vi "SpreadsheetFGV2_Improvements.vi"(0 "Student ID":i32, 1 "FGV Control":T3=enum."Init", 2 "Camera Name":refnum<k21> caption="IMAQdx Session", 11 "Error In":errorcluster) -> (3 "Time Stamp Out":timestamp, 4 "Message":string, 6 "Names":string[](array[string]), 8 "Output 2D Data":string[][](array[string]), 10 "Checked In?":bool, 12 "Cat Points":i32, 13 "Image Out":T1(plugin-control), 14 "Elapsed Time":dbl, 15 "Error Out":errorcluster)   [LabVIEW 2013]
uses:
  Controls/CSVFGVStates.ctl
  <vilib>/userdefined/High Color/IMAQdx.ctl
  Controls/SpreadsheetColumns.ctl
  <vilib>/Utility/file.llb/Write To Spreadsheet File (string).vi
  <vilib>/Utility/file.llb/Read From Spreadsheet File (string).vi
  <vilib>/vision/driver/NI_Vision_Acquisition_Software.lvlib
panel:
  out "Session Out":T2
  out "Checked In":string
  out "all rows":string[][](array[string])
  in  "Replacement":string
  in  "Student Names":i32(listbox)
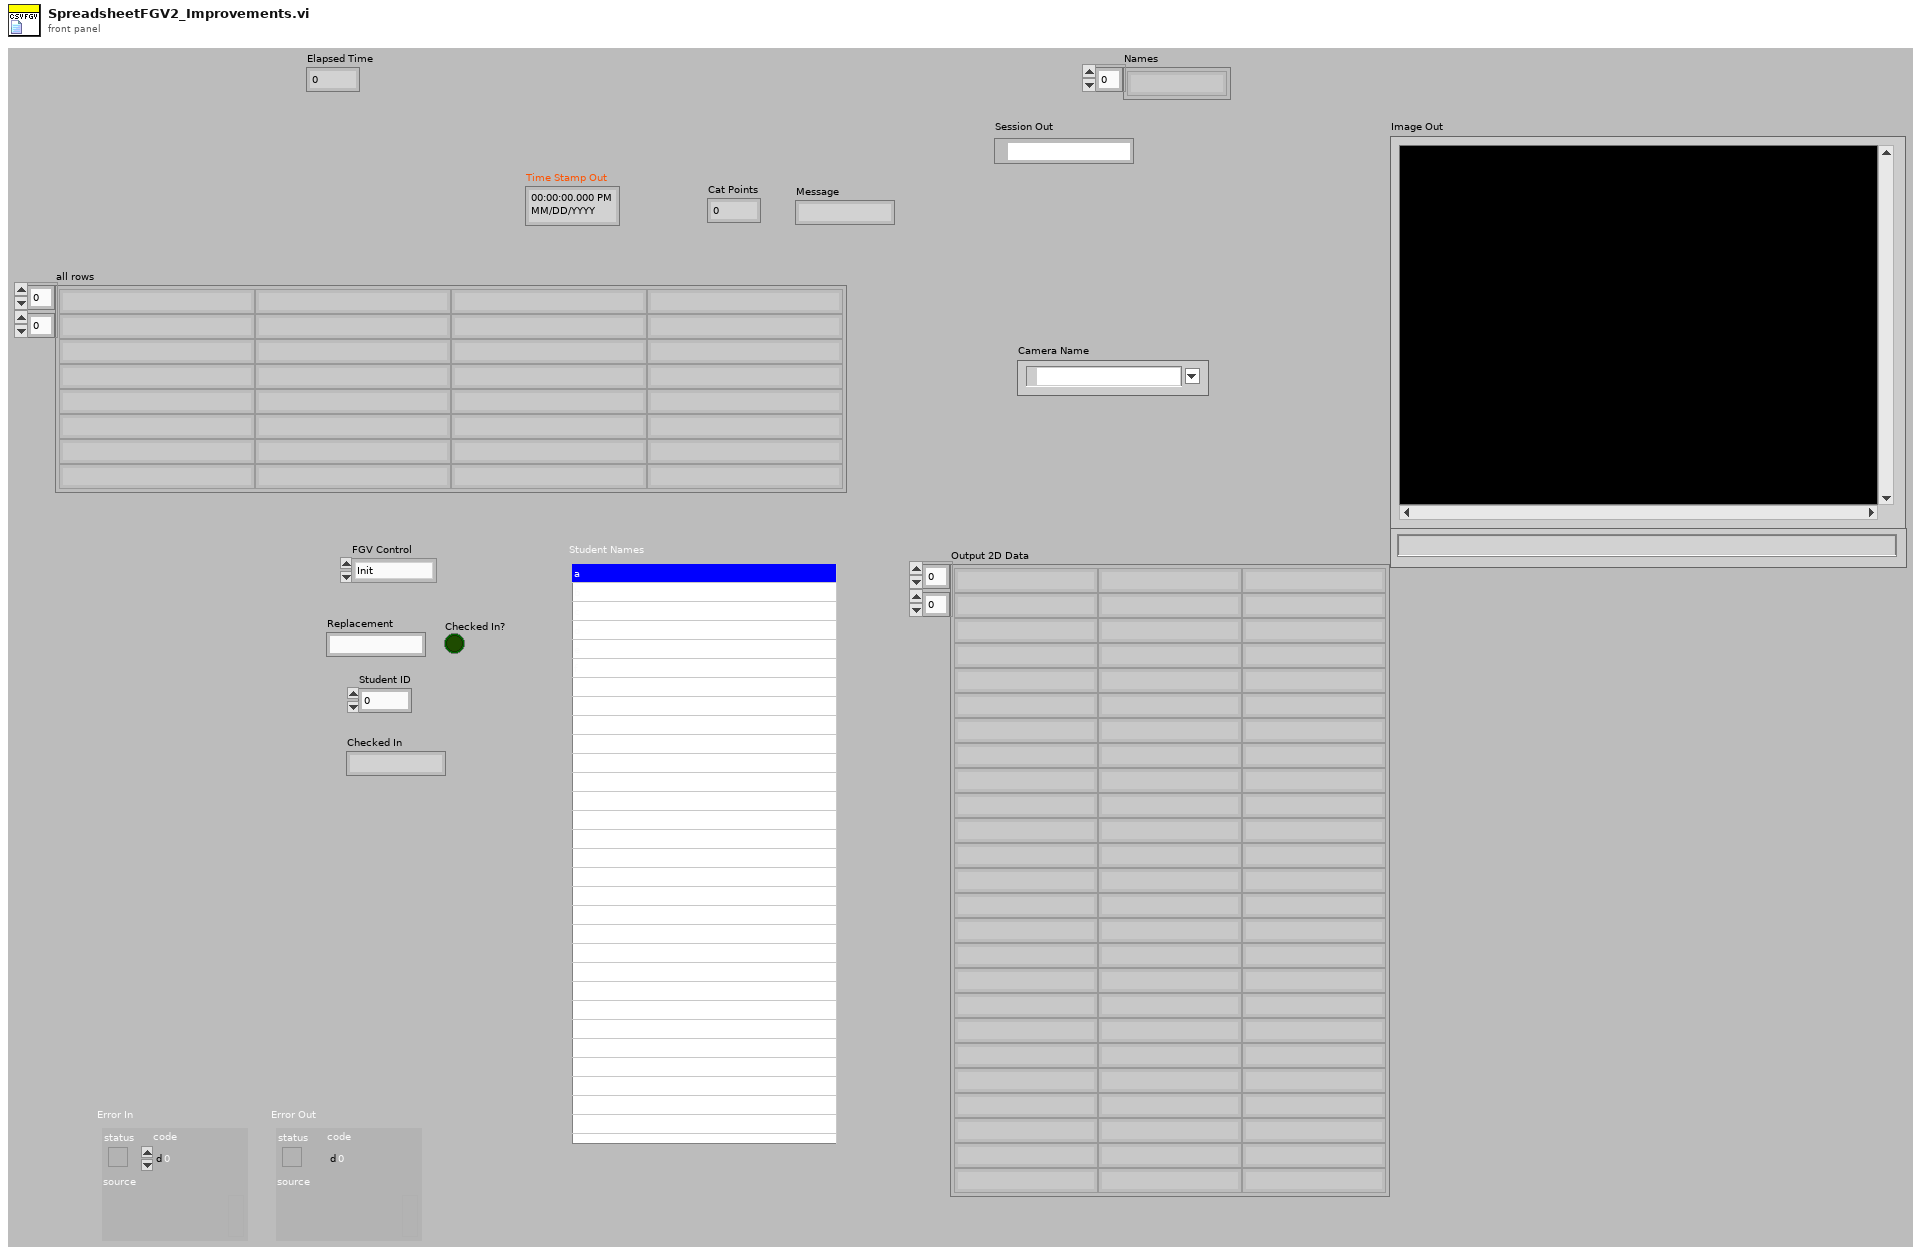
[diagram p1: front panel]
types:
  T1 = typedef "IMAQ Image.ctl" = refnum<image>
  T2 = typedef "IMAQdx.ctl" = refnum<k21>
  T3 = typedef "CSVFGVStates.ctl" = enum16{"Quit", "Init", "Sort", "Check In", "Check Out", "Check Status", "Read CSV", "Close Out"}
  T4 = typedef "SpreadsheetColumns.ctl" = enum16{"Email", "CheckIn", "CheckOut", "Checkin Flag", "Hours", "Minutes", "Seconds", "Total Seconds", "Cat Points"}
  T5 = cluster{"Checkin Flag":T4, "Check In":T4, "Hours":T4, "Minutes":T4, "Seconds":T4, "Check Out":T4, "Email":T4, "Total Seconds":T4}
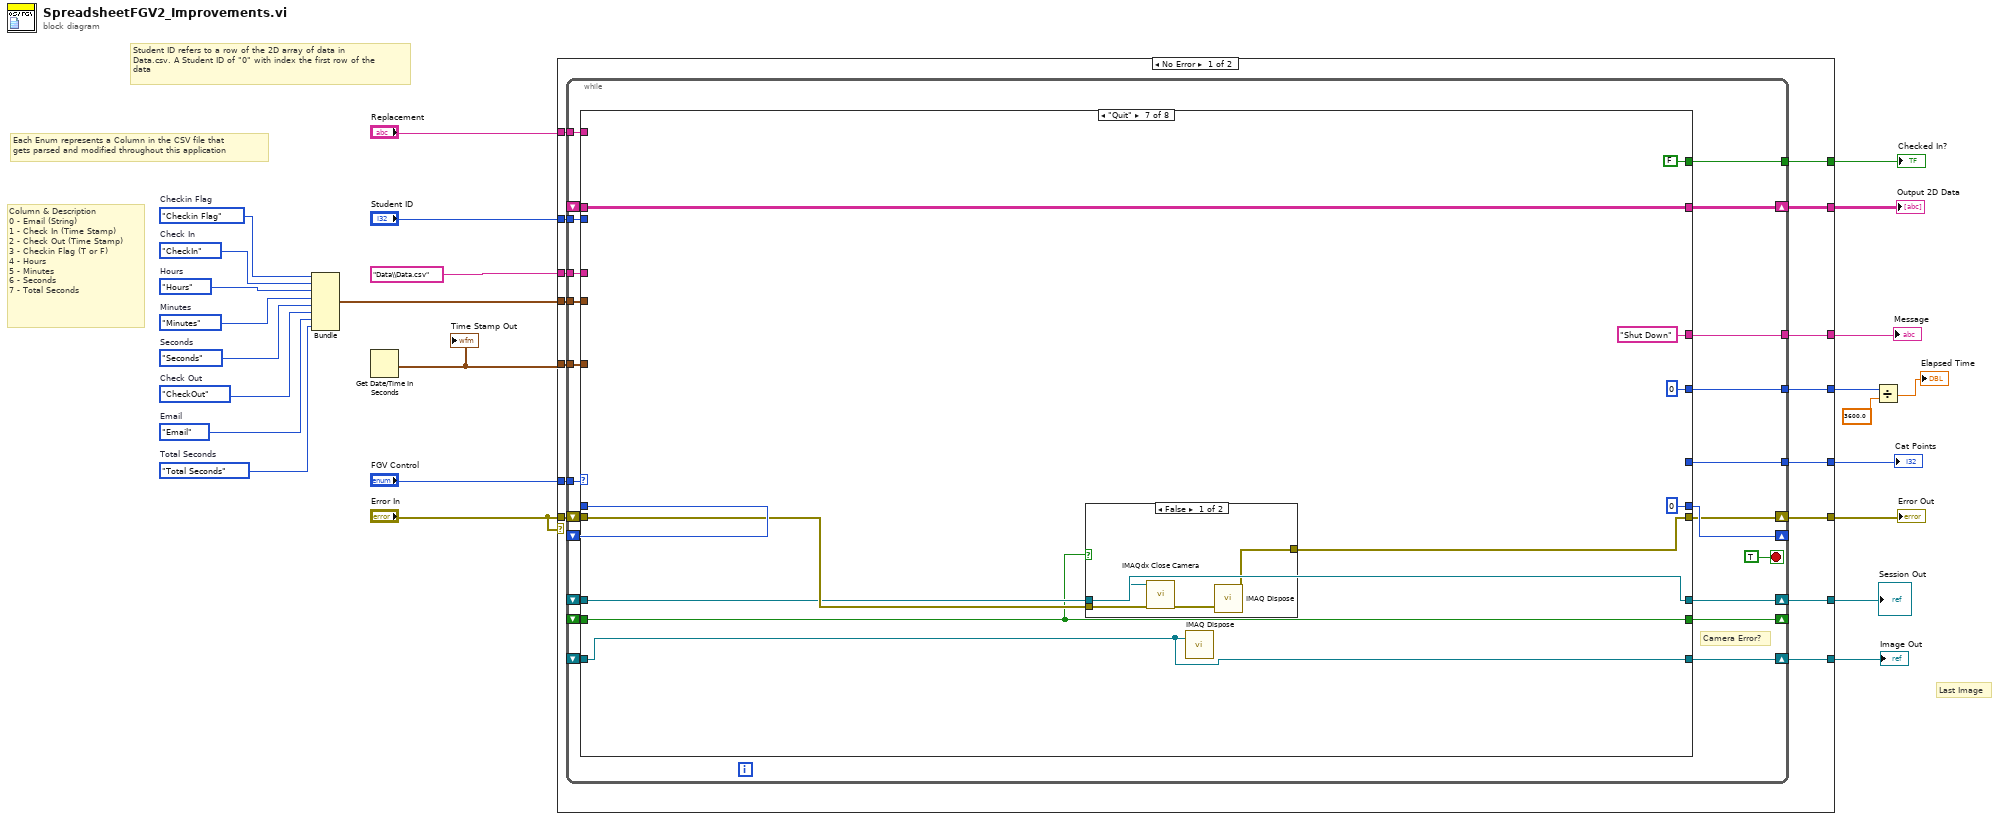
[diagram p0: block diagram]
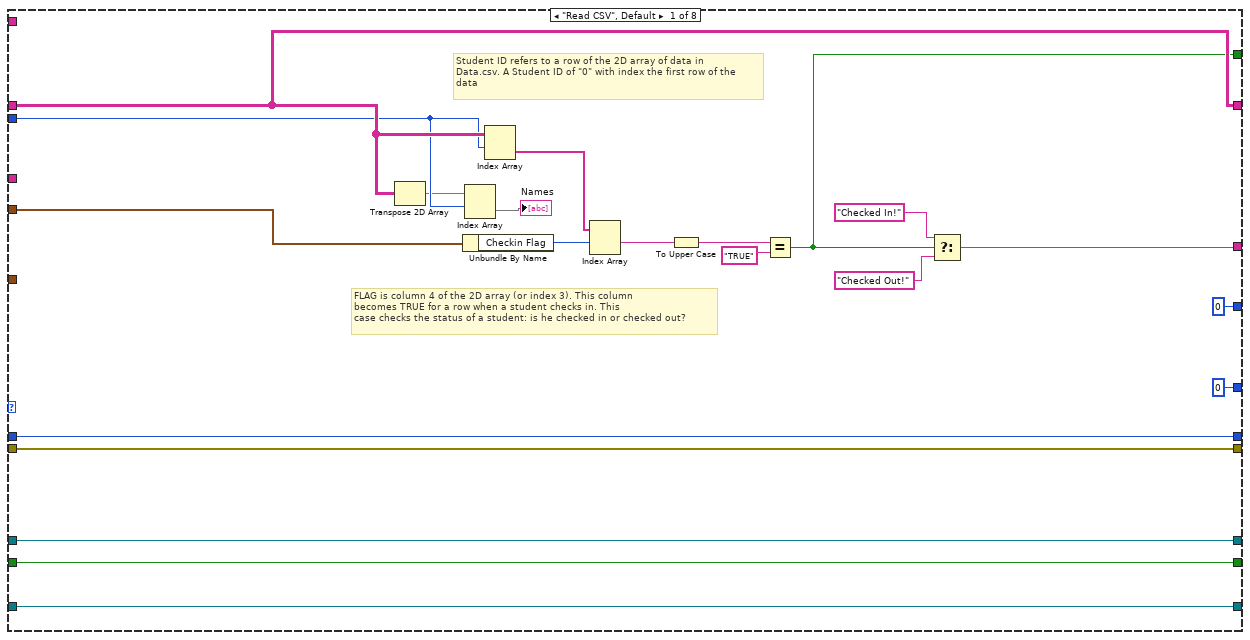
[diagram p2: hidden frame]
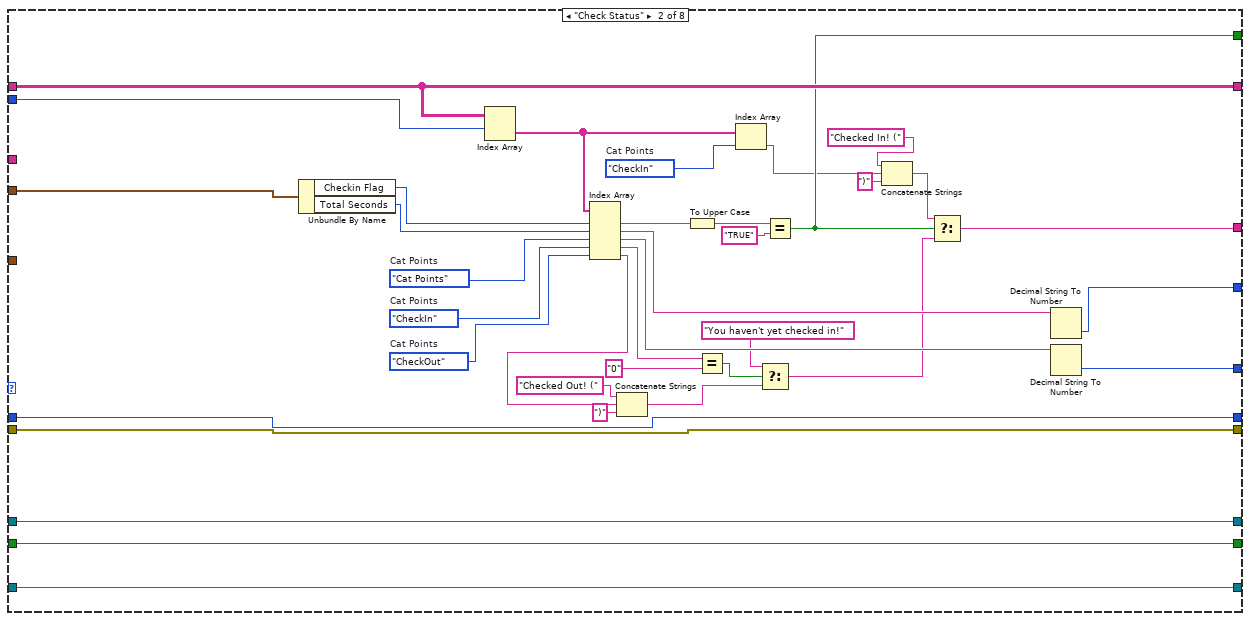
[diagram p3: hidden frame]
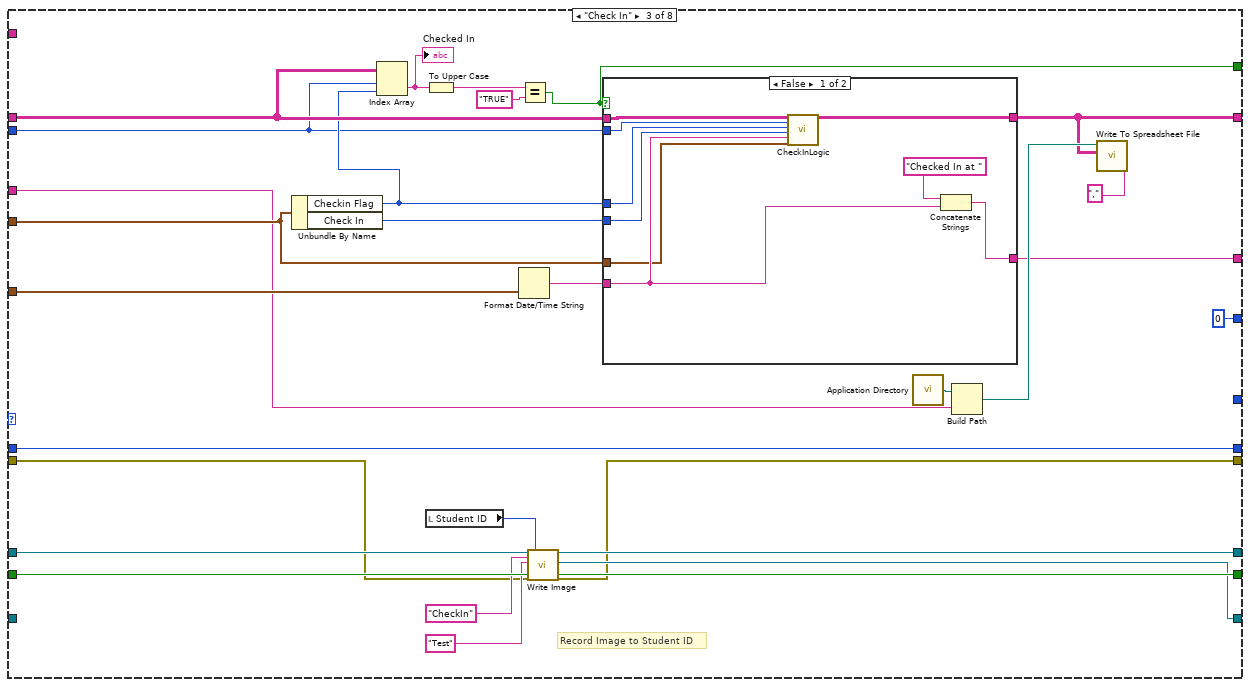
[diagram p4: hidden frame]
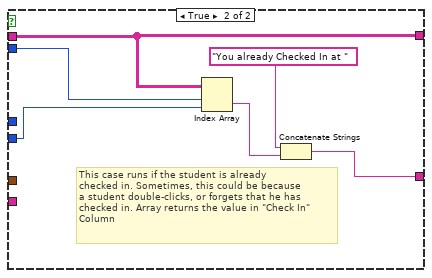
[diagram p5: hidden frame]
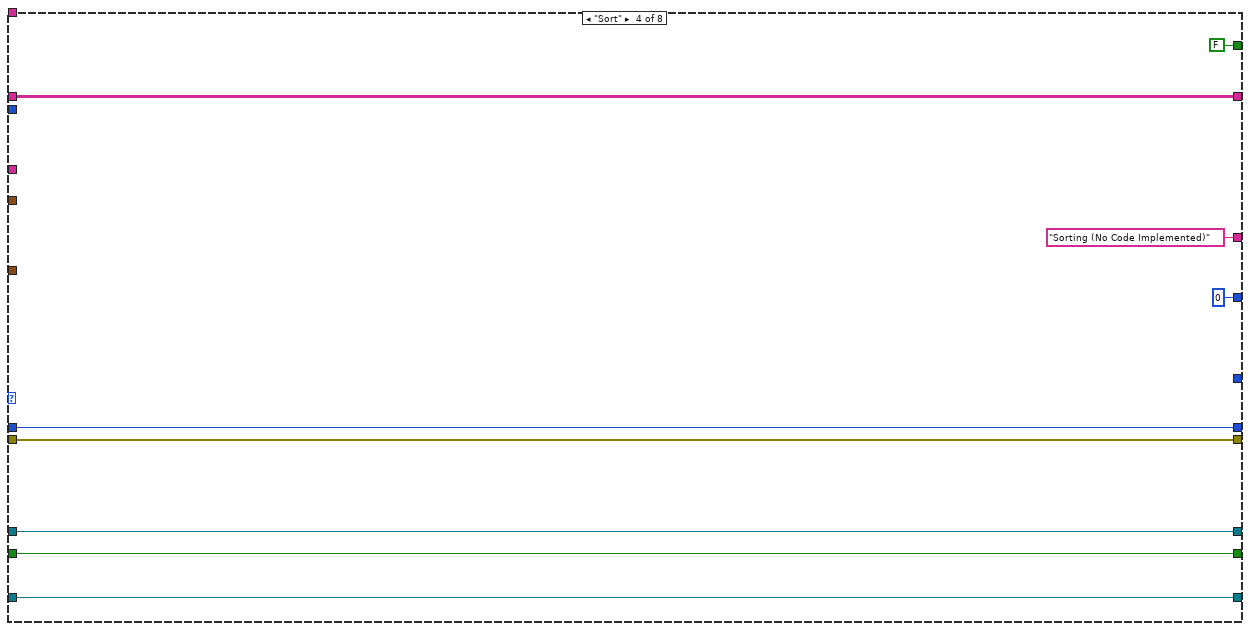
[diagram p6: hidden frame]
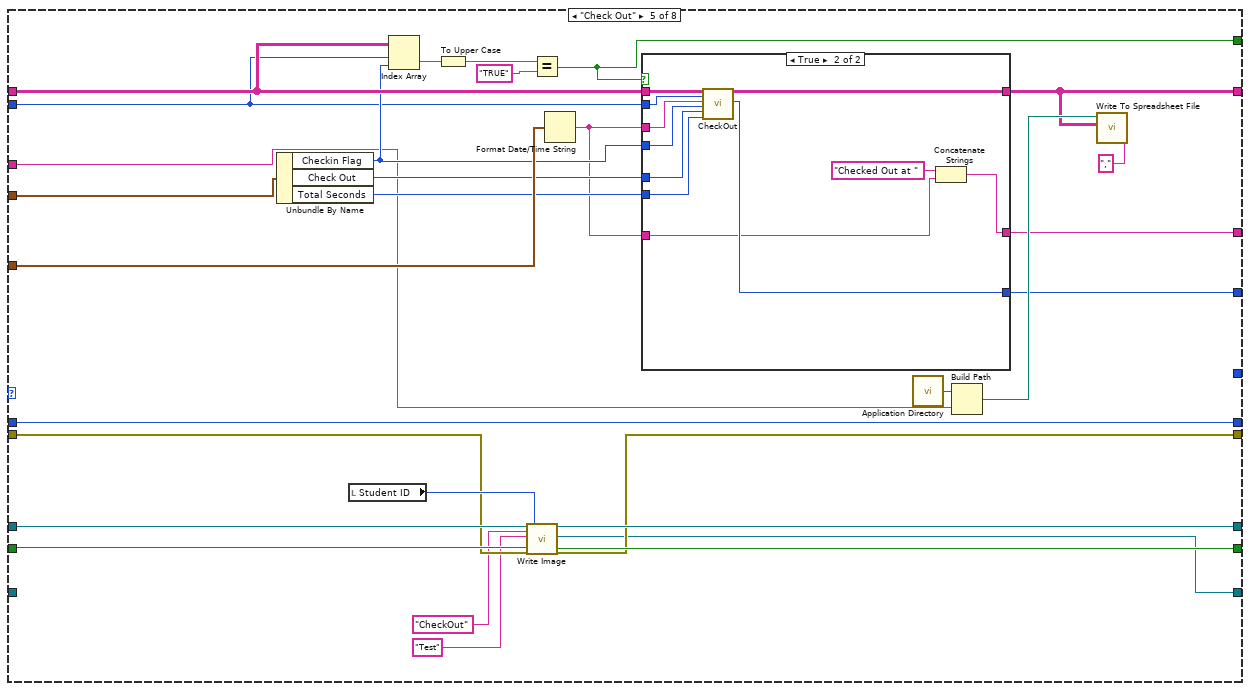
[diagram p7: hidden frame]
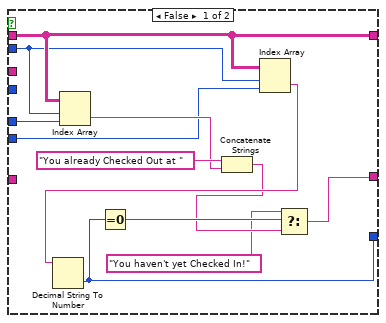
[diagram p8: hidden frame]
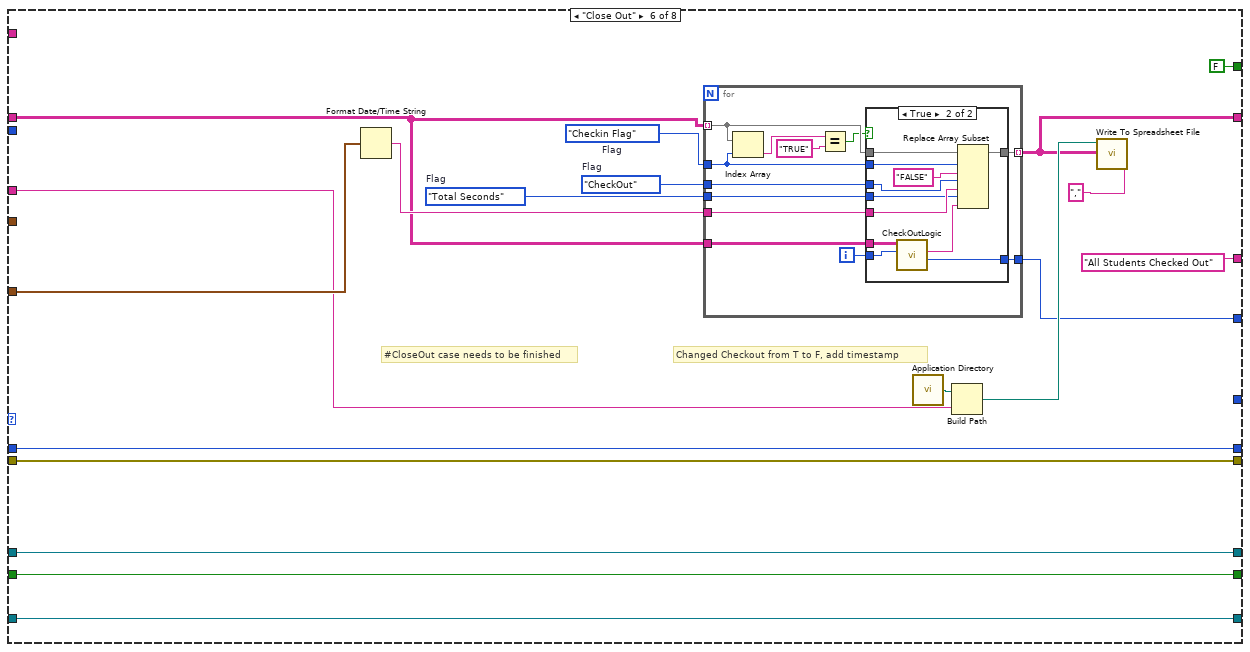
[diagram p9: hidden frame]
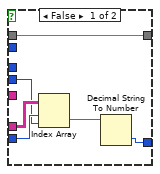
[diagram p10: hidden frame]
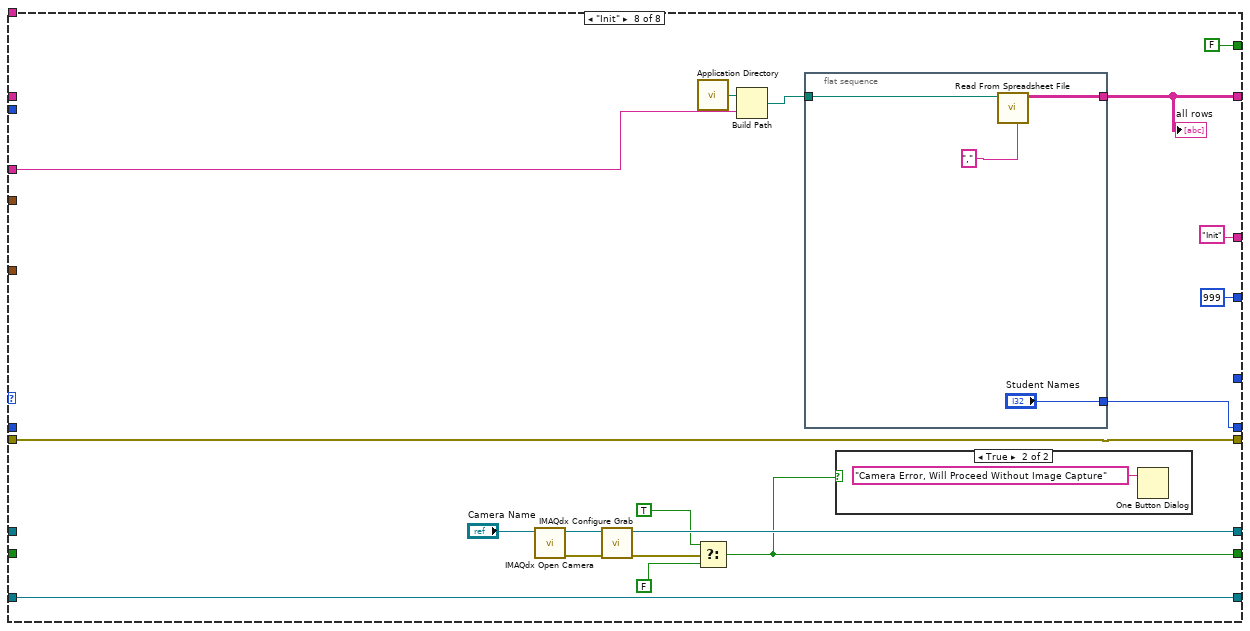
[diagram p12: hidden frame]
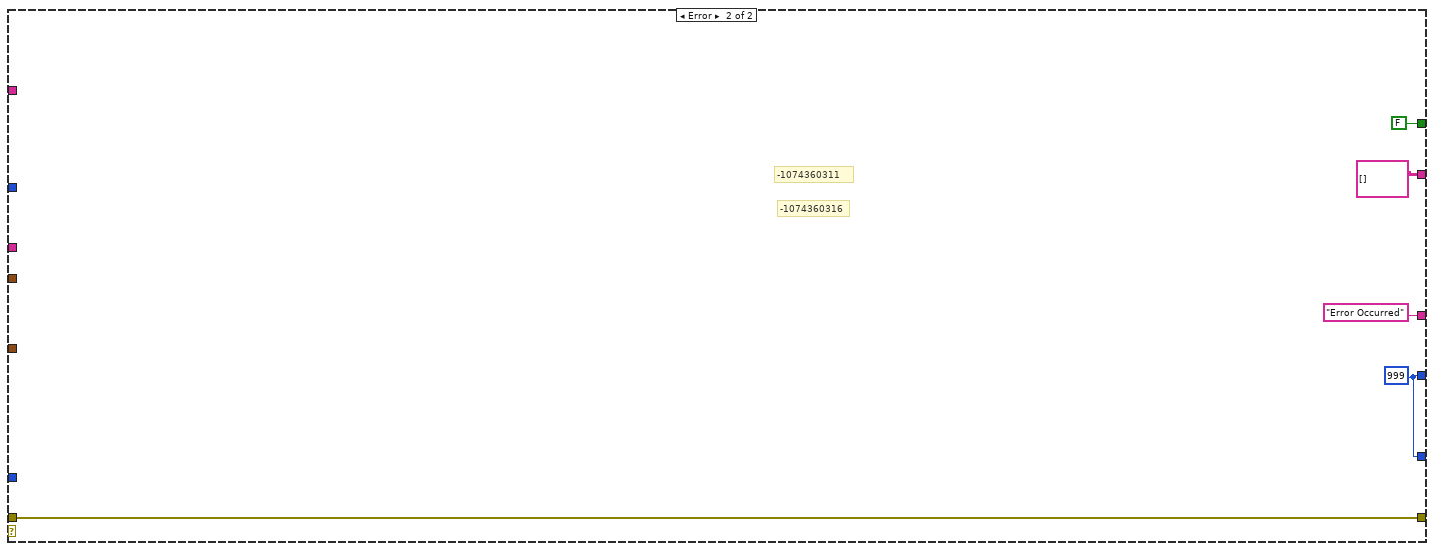
[diagram p14: hidden frame]
diagram:
  w10 = SpreadsheetColumns."Total Seconds"  # Total Seconds
  w11 = SpreadsheetColumns."Email"  # Email
  w12 = SpreadsheetColumns."CheckOut"  # Check Out
  w14 = SpreadsheetColumns."Seconds"  # Seconds
  w15 = SpreadsheetColumns."Minutes"  # Minutes
  w16 = SpreadsheetColumns."Hours"  # Hours
  w18 = SpreadsheetColumns."Checkin Flag"  # Checkin Flag
  w17 = SpreadsheetColumns."CheckIn"  # Check In
  # "Student ID refers to a row of the 2D array of data in \nData.csv. A Student ID of \"0\" with index the first row of the\ndata"
  # "Each Enum represents a Column in the CSV file that\ngets parsed and modified throughout this application"
  # "Last Image"
  # "Column & Description\n0 - Email (String)\n1 - Check In (Time Stamp)\n2 - Check Out (Time Stamp)\n3 - Checkin Flag (T or F)\n4 - Hours\n5 - Minutes\n6 - Seconds\n7 - Total Seconds"
  n1 = Bundle("Checkin Flag"=w18, "Check In"=w17, "Hours"=w16, "Minutes"=w15, "Seconds"=w14, "Check Out"=w12, "Email"=w11, "Total Seconds"=w10) -> (w13:T5)  [unwired: 1 in]
  n2 = Get Date/Time In Seconds() -> (seconds since 1Jan1904=w7:timestamp)
  "Time Stamp Out" <- w7
  n3 = case shown="No Error" "Error In" {
    tunnel: "FGV Control" -> [w40 _]
    tunnel: "Error In" -> [w38 w312]
    tunnel: [w39 w312] -> w23
    tunnel: "Student ID" -> [w37 _]
    tunnel: w7 -> [w36 _]
    tunnel: "Replacement" -> [w35 _]
    tunnel: [w34 FALSE] -> w9
    tunnel: [w33 string[][] [] ("all rows")] -> w20
    tunnel: [w32 "Error Occurred" ("date/time string")] -> w19
    tunnel: [w31 w313] -> w4
    tunnel: w13 -> [w30 _]
    tunnel: "Data\\Data.csv" ("name or relative path") -> [w29 _]
    tunnel: [w28 w313] -> w6
    tunnel: [w27 _] -> w2
    tunnel: [w26 _] -> w1
    frame No Error {
      n4 = while {
        shift-right: [w54] -> w33
        shift-left: _ -> [w49]
        tunnel: w40 -> [w62]
        shift-right: [w61] -> _
        shift-left: _ -> [w60]
        shift-right: [w59] -> w39
        shift-left: w38 -> [w58]
        tunnel: w37 -> [w57]
        tunnel: w36 -> [w56]
        tunnel: w35 -> [w55]
        tunnel: [w53] -> w34
        tunnel: [w52] -> w32
        tunnel: [w51] -> w31
        tunnel: w30 -> [w50]
        tunnel: w29 -> [w48]
        tunnel: [w47] -> w28
        shift-right: [w46] -> w27
        shift-left: _ -> [w45]
        shift-right: [w44] -> w26
        shift-left: _ -> [w43]
        shift-right: [w42] -> _
        shift-left: _ -> [w41]
        stop <- TRUE stop-if-true
        # "Camera Error?"
        n5 = case shown="\"Quit\"" w62 {
          tunnel: w49 -> [w74 w115 w138 w168 w193 w230 w283 _]
          tunnel: [w83 w120 w147 w172 w200 w241 0 ("Student Names") w305] -> w61
          tunnel: w60 -> [w83 w120 w147 w172 w200 w241 _ _]
          tunnel: [w84 w121 w122 w173 w177 w243 w278 w293] -> w59
          tunnel: w58 -> [w84 w121 w123 w173 w178 w243 w277 w293]
          tunnel: w57 -> [w73 w111 w131 _ w183 _ _ _]
          tunnel: w56 -> [_ _ w140 _ w198 w239 _ _]
          tunnel: w55 -> [_ _ _ _ _ _ _ _]
          tunnel: [w74 w115 w133 w168 w197 w238 w283 w299] -> w54
          tunnel: [w70 w112 w137 FALSE w187 FALSE FALSE FALSE] -> w53
          tunnel: [w75 w116 w141 "Sorting (No Code Implemented)" ("date/time string") w192 "All Students Checked Out" ("date/time string") "Shut Down" ("date/time string") "Init" ("date/time string")] -> w52
          tunnel: [0 ("Elapsed Seconds") w108 0 ("Elapsed Seconds") 0 ("Elapsed Seconds") w191 w229 0 ("Elapsed Seconds") 999 ("Elapsed Seconds")] -> w51
          tunnel: w50 -> [w69 w114 w136 _ w190 _ _ _]
          tunnel: w48 -> [_ _ w135 _ w185 w234 _ w300]
          tunnel: [0 w105 _ _ _ _ _ _] -> w47
          tunnel: [w66 w87 w125 w167 w180 w228 w276 w295] -> w46
          tunnel: w45 -> [w66 w87 w130 w167 w181 w228 w276 _]
          tunnel: [w65 w86 w124 w166 w176 w227 w274 w294] -> w44
          tunnel: w43 -> [w65 w86 _ w166 _ w227 w274 w294]
          tunnel: [w64 w85 w129 w165 w179 w226 w275 w289] -> w42
          tunnel: w41 -> [w64 w85 w129 w165 w179 w226 w275 _]
          frame "Read CSV", Default {
            # "FLAG is column 4 of the 2D array (or index 3). This column\nbecomes TRUE for a row when a student checks in. This\ncase checks the status of a student: is he checked in or checked out?"
            # "Student ID refers to a row of the 2D array of data in \nData.csv. A Student ID of \"0\" with index the first row of the\ndata"
            n6 = Transpose 2D Array(2D array=w74) -> (transposed array=w72:string[][])
            n7 = Unbundle By Name(w69) -> ("Checkin Flag"=w68:T4)
            n8 = Index Array(array=w72, index (row)=w73) -> (element=→"Names":string[])  [unwired: 1 in]
            n9 = Index Array(array=w74, index (row)=w73) -> (element=w78:string[])  [unwired: 1 in]
            n10 = Index Array(array=w78, index #1=w68) -> (element #1=w81:string)  [unwired: 1 in, 1 out]
            n11 = To Upper Case(1:w81) -> (0:w80:string)
            n12 = Equal?(x=w80, y="TRUE") -> (x = y?=w70:bool)
            n13 = Select(t="Checked In!" ("y"), s=w70, f="Checked Out!" ("y")) -> (s? t:f=w75:string)
          }
          frame "Check Status" {
            w93 = SpreadsheetColumns."CheckIn"  # Cat Points
            w92 = SpreadsheetColumns."CheckOut"  # Cat Points
            w104 = SpreadsheetColumns."CheckIn"  # Cat Points
            w107 = SpreadsheetColumns."Cat Points"  # Cat Points
            n14 = Unbundle By Name(w114) -> ("Checkin Flag"=w113:T4, "Total Seconds"=w110:T4)
            n15 = Index Array(array=w115, index (row)=w111) -> (element=w94:string[])  [unwired: 1 in]
            n16 = Index Array(array=w94, index #1=w113, index #2=w110, index #3=w107, index #4=w104, index #5=w92) -> (element #1=w119:string, element #2=w109:string, element #3=w106:string, element #4=w103:string, element #5=w96:string)
            n17 = Concatenate Strings("Checked Out! (" ("y"), w96, ")" ("string")) -> (w97:string)
            n18 = To Upper Case(1:w119) -> (0:w118:string)
            n19 = Equal?(x=w103, y="0") -> (x = y?=w101:bool)
            n20 = Index Array(array=w94, index=w93) -> (element=w90:string)
            n21 = Select(t="You haven't yet checked in!", s=w101, f=w97) -> (s? t:f=w100:string)
            n22 = Equal?(x=w118, y="TRUE") -> (x = y?=w112:bool)
            n23 = Concatenate Strings("Checked In! (" ("y"), w90, ")" ("string")) -> (w88:string)
            n24 = Select(t=w88, s=w112, f=w100) -> (s? t:f=w116:string)
            n25 = Decimal String To Number(string=w109) -> (number=w108:i32)  [unwired: 2 in, 1 out]
            n26 = Decimal String To Number(string=w106) -> (number=w105:i32)  [unwired: 2 in, 1 out]
          }
          frame "Check In" {
            # "Record Image to Student ID"
            n27 = Unbundle By Name(w136) -> ("Checkin Flag"=w134:T4, "Check In"=w139:T4)
            n28 = Index Array(array=w138, index (row)=w131, index (col)=w134) -> (element=w144:string)
            "Checked In" <- w144
            n29 = To Upper Case(1:w144) -> (0:w143:string)
            n30 = local read "Student ID"() -> (w128:i32)
            n31 = Format Date/Time String(seconds (now)=w140) -> (date/time string=w145:string)  [unwired: 2 in]
            n32 = Equal?(x=w143, y="TRUE") -> (x = y?=w137:bool)
            n33 = call "Write Image.vi"("Session In"=w130, "Folder"="CheckIn", "Temp Image Name"="Test" ("Image Name"), "Camera Missing?"=w129, "Error In"=w123, "Student ID"=w128) -> ("Session Out"=w125:T2, "Image Out"=w124:T1, "Error Out"=w122:errorcluster)  [unwired: 11 in]
            n34 = case shown="False" w137 {
              tunnel: w145 -> [w151 _]
              tunnel: [w155 w164] -> w133
              tunnel: w131 -> [w154 w163]
              tunnel: w138 -> [w156 w164]
              tunnel: [w157 w160] -> w141
              tunnel: w134 -> [w153 _]
              tunnel: w139 -> [w152 w159]
              tunnel: w136 -> [w150 _]
              frame False {
                n35 = call "CheckInLogic.vi"("all rows in"=w156, "Student ID"=w154, "Checkin Flag"=w153, "Check In"=w152, "date/time string"=w151, "Time Cluster"=w150) -> ("all rows out"=w155:string[][])  [unwired: 13 in]
                n36 = Concatenate Strings("Checked In at " ("String"), w151) -> (w157:string)
              }
              frame True {
                # "This case runs if the student is already \nchecked in. Sometimes, this could be because\na student double-clicks, or forgets that he has \nchecked in. Array returns the value in \"Check In\" \nColumn"
                n37 = Index Array(array=w164, index (row)=w163, index (col)=w159) -> (element=w161:string)
                n38 = Concatenate Strings("You already Checked In at " ("delimiter (\\t)"), w161) -> (w160:string)
              }
            }
            n39 = call <vilib>:"Application Directory.vi"() -> ("Application Directory"=w149:path)
            n40 = Build Path(base path=w149, name or relative path=w135) -> (appended path=w148:path)
            n41 = call-poly <vilib>:"Write To Spreadsheet File.vi"("delimiter (\\t)"="," ("delimiter (\\t)"), "2D data"=w133, "file path (dialog if empty)"=w148) -> ()  [unwired: 5 in, 1 out]
          }
          frame "Sort" {
          }
          frame "Check Out" {
            n42 = Unbundle By Name(w190) -> ("Checkin Flag"=w186:T4, "Check Out"=w188:T4, "Total Seconds"=w189:T4)
            n43 = local read "Student ID"() -> (w182:i32)
            n44 = Index Array(array=w193, index (row)=w183, index (col)=w186) -> (element=w196:string)
            n45 = To Upper Case(1:w196) -> (0:w195:string)
            n46 = call "Write Image.vi"("Session In"=w181, "Folder"="CheckOut", "Temp Image Name"="Test" ("Image Name"), "Camera Missing?"=w179, "Error In"=w178, "Student ID"=w182) -> ("Session Out"=w180:T2, "Image Out"=w176:T1, "Error Out"=w177:errorcluster)  [unwired: 11 in]
            n47 = Equal?(x=w195, y="TRUE") -> (x = y?=w187:bool)
            n48 = Format Date/Time String(seconds (now)=w198) -> (date/time string=w184:string)  [unwired: 2 in]
            n49 = case shown="True" w187 {
              tunnel: [w211 w222] -> w197
              tunnel: w183 -> [w210 w221]
              tunnel: w193 -> [w211 w223]
              tunnel: [w204 w225] -> w192
              tunnel: [w207 w216] -> w191
              tunnel: w189 -> [w209 w219]
              tunnel: w188 -> [w212 w220]
              tunnel: w186 -> [_ w218]
              tunnel: w184 -> [_ w217]
              tunnel: w184 -> [_ w215]
              frame False {
                n50 = Index Array(array=w211, index (row)=w210, index (col)=w212) -> (element=w213:string)
                n51 = Concatenate Strings("You already Checked Out at " ("string"), w213) -> (w205:string)
                n52 = Index Array(array=w211, index (row)=w210, index (col)=w209) -> (element=w208:string)
                n53 = Decimal String To Number(string=w208) -> (number=w207:i32)  [unwired: 2 in, 1 out]
                n54 = Equal To 0?(x=w207) -> (x = 0?=w206:bool)
                n55 = Select(t="You haven't yet Checked In!", s=w206, f=w205) -> (s? t:f=w204:string)
              }
              frame True {
                n56 = call "CheckOut.vi"("Student List In"=w223, "Student ID"=w221, "date/time string"=w217, "Checkin Flag"=w218, "Check Out"=w220, "Total Seconds"=w219) -> ("Student List Out"=w222:string[][], "Total Elapsed Time"=w216:i32)  [unwired: 12 in]
                n57 = Concatenate Strings("Checked Out at " ("string"), w215) -> (w225:string)
              }
            }
            n58 = call <vilib>:"Application Directory.vi"() -> ("Application Directory"=w202:path)
            n59 = Build Path(base path=w202, name or relative path=w185) -> (appended path=w201:path)
            n60 = call-poly <vilib>:"Write To Spreadsheet File.vi"("delimiter (\\t)"="," ("delimiter (\\t)"), "2D data"=w197, "file path (dialog if empty)"=w201) -> ()  [unwired: 5 in, 1 out]
          }
          frame "Close Out" {
            w231 = SpreadsheetColumns."Total Seconds"  # Flag
            w232 = SpreadsheetColumns."CheckOut"  # Flag
            w233 = SpreadsheetColumns."Checkin Flag"  # Flag
            # "#CloseOut case needs to be finished"
            # "Changed Checkout from T to F, add timestamp"
            n61 = Format Date/Time String(seconds (now)=w239) -> (date/time string=w236:string)  [unwired: 2 in]
            n62 = for {
              tunnel: [w256] -> w238 mode=indexing
              tunnel: w230 -> [w249] mode=indexing
              tunnel: w236 -> [w255]
              tunnel: w233 -> [w248]
              tunnel: w232 -> [w254]
              tunnel: w231 -> [w252]
              tunnel: w230 -> [w251]
              tunnel: [w250] -> w229
              i -> [w253]
              n63 = Index Array(array=w249, index=w248) -> (element=w247:string)
              n64 = Equal?(x=w247, y="TRUE") -> (x = y?=w245:bool)
              n65 = case shown="True" w245 {
                tunnel: [w262 w273] -> w256
                tunnel: w255 -> [_ w271]
                tunnel: w254 -> [_ w270]
                tunnel: w253 -> [w260 w269]
                tunnel: w252 -> [w259 w267]
                tunnel: w251 -> [w261 w266]
                tunnel: [w257 w265] -> w250
                tunnel: w249 -> [w262 w264]
                tunnel: w248 -> [_ w263]
                frame False {
                  n66 = Index Array(array=w261, index (row)=w260, index (col)=w259) -> (element=w258:string)
                  n67 = Decimal String To Number(string=w258) -> (number=w257:i32)  [unwired: 2 in, 1 out]
                }
                frame True {
                  n68 = call "CheckOutLogic.vi"("Student ID"=w269, "Student List In"=w266) -> ("Total Elapsed Time"=w265:i32, "Total Seconds Out"=w268:string)  [unwired: 7 in, 1 out]
                  n69 = Replace Array Subset(array=w264, new element #1="FALSE" ("new element/subarray"), index #1=w263, new element #2=w271, index #2=w270, new element #3=w268, index #3=w267) -> (w273:string[])
                }
              }
            }
            n70 = call <vilib>:"Application Directory.vi"() -> ("Application Directory"=w244:path)
            n71 = Build Path(base path=w244, name or relative path=w234) -> (appended path=w242:path)
            n72 = call-poly <vilib>:"Write To Spreadsheet File.vi"("delimiter (\\t)"="," ("delimiter (\\t)"), "2D data"=w238, "file path (dialog if empty)"=w242) -> ()  [unwired: 5 in, 1 out]
          }
          frame "Quit" {
            n73 = case shown="False" w275 {
              tunnel: [w286 w288] -> w278
              tunnel: w277 -> [w285 w288]
              tunnel: w276 -> [w284 _]
              frame False {
                n74 = call <vilib>:"IMAQdx Close Camera.vi"("error in"=w285, "Session In"=w284) -> ("error out"=w287:errorcluster)  [unwired: 9 out]
                n75 = call "IMAQ Dispose"("error in (no error)"=w287) -> ("error out"=w286:errorcluster)  [unwired: 5 in]
              }
              frame True {
              }
            }
            n76 = call "IMAQ Dispose"("Image"=w274) -> ()  [unwired: 5 in, 1 out]
          }
          frame "Init" {
            n77 = call <vilib>:"IMAQdx Open Camera.vi"("Session In"="Camera Name") -> ("error out"=w298:errorcluster, "Session Out"=w297:T2)  [unwired: 2 in, 7 out]
            n78 = call <vilib>:"IMAQdx Configure Grab.vi"("error in"=w298, "Session In"=w297) -> ("error out"=w292:errorcluster, "Session Out"=w295:T2)  [unwired: 8 out]
            n79 = call <vilib>:"Application Directory.vi"() -> ("Application Directory"=w306:path)
            n80 = Select(t=TRUE, s=w292, f=FALSE) -> (s? t:f=w289:bool)
            n81 = Build Path(base path=w306, name or relative path=w300) -> (appended path=w304:path)
            n82 = flat-sequence {
              tunnel: w304 -> [w311]
              tunnel: [w310] -> w299
              tunnel: ["Student Names"] -> w305
              frame #0 {
                n83 = call-poly <vilib>:"Read From Spreadsheet File.vi"("delimiter (\\t)"="," ("delimiter (\\t)"), "file path (dialog if empty)"=w311) -> ("all rows"=w310:string[][])  [unwired: 5 in, 4 out]
              }
            }
            n84 = case shown="True" w289 {
              frame False {
              }
              frame True {
                n85 = One Button Dialog(message="Camera Error, Will Proceed Without Image Capture") -> ()  [unwired: 1 in, 1 out]
              }
            }
            "all rows" <- w299
          }
        }
      }
    }
    frame Error {
      w313 = 999 ("Elapsed Seconds")
      # "-1074360316"
      # "-1074360311"
    }
  }
  "Error Out" <- w23
  "Checked In?" <- w9
  "Output 2D Data" <- w20
  "Message" <- w19
  "Cat Points" <- w6
  "Session Out" <- w2
  "Image Out" <- w1
  n86 = Divide(x=w4, y=3600.0) -> (x/y=→"Elapsed Time":dbl)
